vi "Do.vi"(8 "error in (no error)":errorcluster, 10 "Actor in":refnum<class "Actor.lvclass">, 11 "Set Laser Enable MSG":refnum<class "Set Las Enable MSG.lvclass">) -> (0 "error out":errorcluster, 2 "Actor out":refnum<class "Actor.lvclass">)   [LabVIEW 2014, in "ePAS Library.lvlib" / "Set Las Enable MSG.lvclass"]
doc: "(<B>Filename</B>: Actor Framework.lvlib:Message.lvclass:Do.vi)\n\nDefines what a message does when it is received by an actor. Generally, a message instructs an actor to invoke one of its methods. By default, this method does nothing. A child class must override it to define behavior. Create a child class by using the Actor Framework Message Maker dialog box."
uses:
  Set Las Enable MSG.lvclass
  <vilib>/ActorFramework/Actor/Actor.lvclass
  Instr Actor.lvclass
  PAS/Commands/Copy of Change Laser Enable State/Change Laser Enable State.lvclass
  Set Las Enable MSG.lvclass/Set Las Enable MSG.ctl
  PAS/Commands/Copy of Change Laser Enable State/Change Laser Enable State.lvclass/Change Laser Enable State.ctl
  Controller/Messages/Update CVT/Update CVT Data.lvclass
  Controller/Messages/Update CVT/Update CVT Data.lvclass/Update CVT Data.ctl
  Controller/Messages/Update CVT/Write tag.vi
  Controller/Messages/Update CVT/Write Data.vi
  Controller/Messages/Update CVT/Write Group.vi
  PAS/Commands/Copy of Change Laser Enable State/Write Enabled.vi
  reusable/Command/Command.lvclass
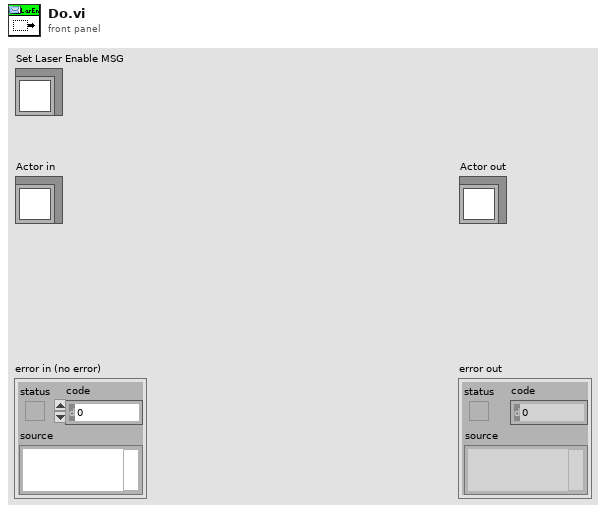
[diagram p1: front panel]
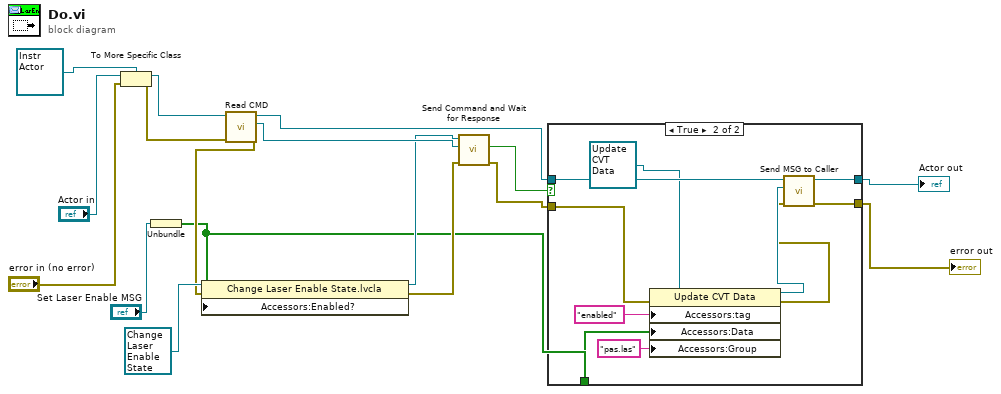
[diagram p0: block diagram]
diagram:
  n1 = To More Specific Class(target class=refnum<class "Instr Actor.lvclass"> refnum ("Instrument Lib:Instr"), reference="Actor in", error in="error in (no error)") -> (specific class reference=w15:refnum<class "Instr Actor.lvclass">, error out=w14:errorcluster)
  n2 = Unbundle("Set Laser Enable MSG") -> (w1:bool[])
  n3 = call "Read CMD.vi"("error in (no error)"=w14, "Instr Actor in"=w15) -> ("error out"=w7:errorcluster, "CMD"=w10:refnum<queue>, "Instr Actor out"=w6:refnum<class "Instr Actor.lvclass">)  [unwired: 7 in]
  n4 = property class="Change Laser Enable State.lvcla"(reference=refnum<class "Change Laser Enable State.lvclass"> refnum ("Change Laser Enable State.lvclass"), error in=w7, "Accessors:Enabled?"=w1) -> (reference out=w9:refnum<class "Change Laser Enable State.lvclass">, error out=w8:errorcluster)
  n5 = call "Send Command and Wait for Response.vi"("error in"=w8, "cmd queue"=w10, "CMD in"=w9) -> ("error out"=w4:errorcluster, "cmd good?"=w5:bool)  [unwired: 6 in, 1 out]
  n6 = case shown="True" w5 {
    tunnel: w1 -> [_ w25]
    tunnel: w6 -> [w19 w29]
    tunnel: [w19 w28] -> w2
    tunnel: w4 -> [w18 w23]
    tunnel: [w18 w27] -> w3
    frame False {
    }
    frame True {
      n7 = property class="Update CVT Data"(reference=refnum<class "Update CVT Data.lvclass"> refnum ("Controller.lvlib:Update CVT Data"), error in=w23, "Accessors:tag"="enabled" ("Key"), "Accessors:Data"=w25, "Accessors:Group"="pas.las" ("Group")) -> (reference out=w24:refnum<class "Update CVT Data.lvclass">, error out=w22:errorcluster)
      n8 = call "Send MSG to Caller.vi"("error in"=w22, "Message"=w24, "Instr in"=w29) -> ("error out"=w27:errorcluster, "Instr out"=w28:refnum<class "Instr Actor.lvclass">)  [unwired: 7 in]
    }
  }
  "error out" <- w3
  "Actor out" <- w2
